vi "_Remote Connect.vi"(4 "error in (no error)":errorcluster, 7 "IP Address":string) -> (0 "error out":errorcluster, 3 "TCP":bool)   [LabVIEW 2015]
uses:
  Type/_RT Command.ctl
  Configuration/_Global Configuration.vi
  <vilib>/Utility/config.llb/Write Key (String).vi
  <vilib>/Utility/config.llb/NI_LVConfig.lvlib
panel:
  out "Info":string
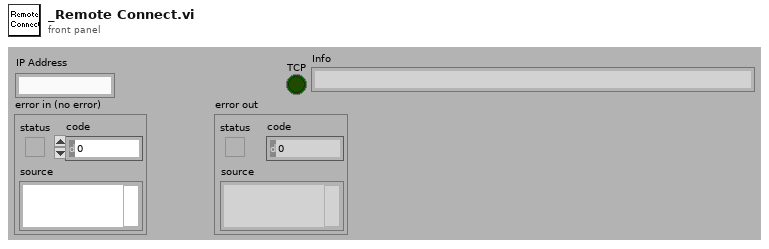
[diagram p1: front panel]
types:
  T1 = typedef "NI_LVConfig.lvlib/Config Data RefNum.ctl" = refnum<k1>
  T2 = typedef "_RT Command.ctl" = enum16{"xml Start Run", "xml Start Actual Run", "xml Stop Run", "xml Runtime Update", "xml Get Status", "xml Get Table", "xml Set Table", "xml Get Configuration", "xml System Status", "xml Set LC Input Logic", "xml Get Data", "xml Get Info", "Start", "StartActualRun", "Stop", "Runtime Update", "Get Data", "Get Info", "Get Status", "Get Param", "Get Config", "Get Table", "Read ADC", "Set Oscillator", "Update Config", "Update Table", "Set All Pol", "Set Pol and DC", "Set Max Mass", "Toggle RP", "Toggle EL", "Set PIC", "Initialize Turbo", "Send Turbo Comm", "Close Turbo", "P1", "P2", "P3", "Send Serial", "Set LC Out", "Get LC In", "Read VAC", "Test Table", "Toggle Power", "Get Startup", "Set Startup", "Get ADC Table", "Set ADC Table", "Get Brief Status", "Get Detail Status", "Auxiliary Update", "Set CC Logics", "Set CC Input Logics", "Ignore Error", "invalid"}
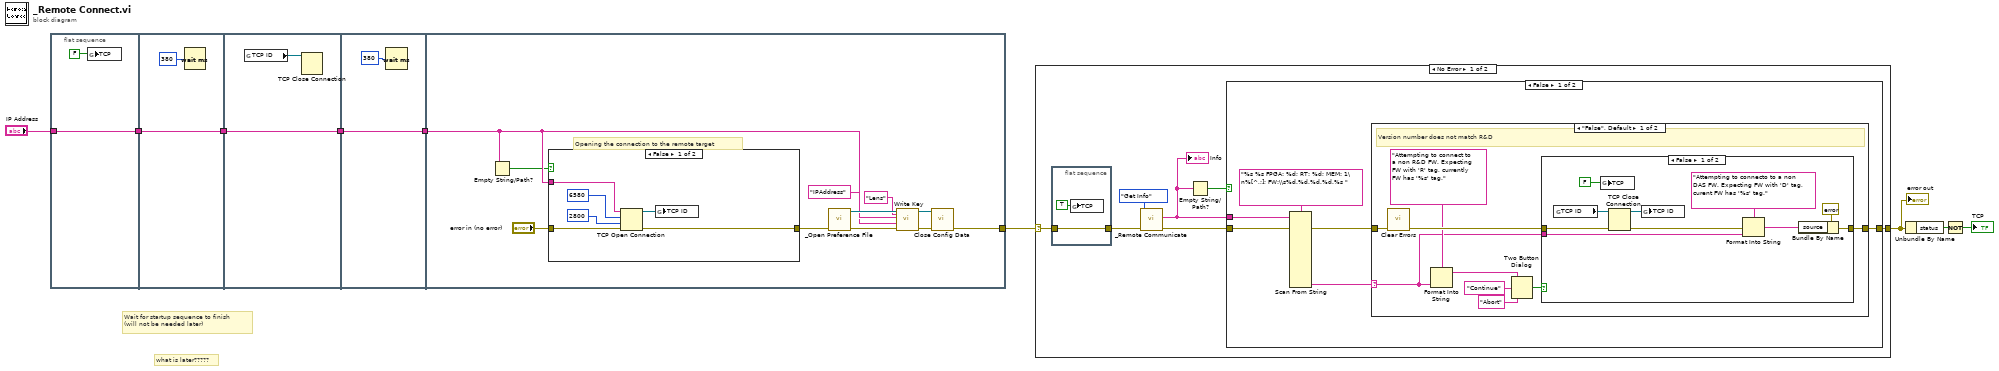
[diagram p0: block diagram]
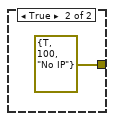
[diagram p2: hidden frame]
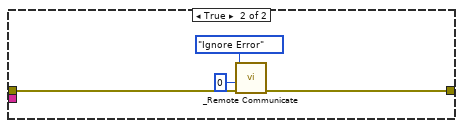
[diagram p3: hidden frame]
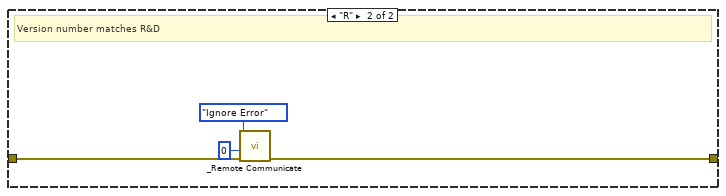
[diagram p4: hidden frame]
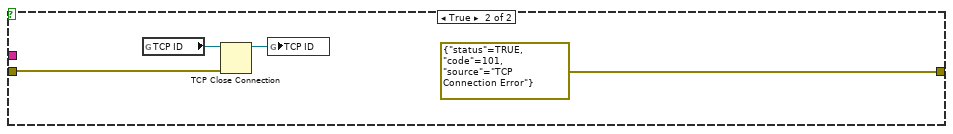
[diagram p5: hidden frame]
diagram:
  # "what is later?????"
  # "Wait for startup sequence to finish\n(will not be needed later)"
  n1 = flat-sequence {
    tunnel: "IP Address" -> [w10]
    tunnel: [w10] -> w4
    tunnel: w4 -> [w12]
    tunnel: [w12] -> w3
    tunnel: w3 -> [w14]
    tunnel: [w14] -> w2
    tunnel: w2 -> [w16]
    tunnel: [w16] -> w1
    tunnel: [w20] -> w9
    tunnel: w1 -> [w22]
    frame #0 {
      n2 = global write "_Global Configuration.vi" "TCP"(FALSE ("TCP")) -> ()
    }
    frame #1 {
      n3 = Wait (ms)(milliseconds to wait=u32 380) -> ()  [unwired: 1 out]
    }
    frame #2 {
      n4 = global read "_Global Configuration.vi" "TCP ID"() -> (w15:refnum<k5>)
      n5 = TCP Close Connection(connection ID=w15) -> ()  [unwired: 1 in, 3 out]
    }
    frame #3 {
      n6 = Wait (ms)(milliseconds to wait=u32 380) -> ()  [unwired: 1 out]
    }
    frame #4 {
      # "Opening the connection to the remote target"
      n7 = Empty String/Path?(string/path=w22) -> (empty?=w19:bool)
      n8 = case shown="False" w19 {
        tunnel: w22 -> [w33 _]
        tunnel: "error in (no error)" -> [w34 _]
        tunnel: [w30 errorcluster {"status"=TRUE, "code"=100, "source"="No IP"} ("error out")] -> w21
        frame False {
          n9 = TCP Open Connection(address=w33, remote port or service name=u16 6580 ("remote port"), timeout ms (60000)=2800, error in (no error)=w34) -> (connection ID=w31:refnum<k5>, error out=w30:errorcluster)  [unwired: 1 out]
          n10 = global write "_Global Configuration.vi" "TCP ID"(w31) -> ()
        }
        frame True {
        }
      }
      n11 = call "_Open Preference File.vi"("error In"=w21) -> ("error"=w26:errorcluster, "refnum"=w25:T1)  [unwired: 2 in, 3 out]
      n12 = call-poly <vilib>:"Write Key.vi"("section"="Lens", "error in (no error)"=w26, "value"=w22, "key"="IPAddress" ("section"), "refnum"=w25) -> ("error out"=w28:errorcluster, "refnum out"=w27:T1)  [unwired: 1 in, 4 out]
      n13 = call <vilib>:"Close Config Data.vi"("error in (no error)"=w28, "refnum"=w27) -> ("error out"=w20:errorcluster)  [unwired: 1 in, 8 out]
    }
  }
  n14 = case shown="No Error" w9 {
    selector: w9 -> [w41 w82]
    tunnel: [w38 w82] -> w7
    frame No Error {
      n15 = flat-sequence {
        tunnel: w41 -> [w80]
        tunnel: [w80] -> w40
        frame #0 {
          n16 = global write "_Global Configuration.vi" "TCP"(TRUE) -> ()
        }
      }
      n17 = call "_Remote Communicate.vi"("error in (no error)"=w40, "Command"=_RT_Command."Get Info") -> ("error out"=w39:errorcluster, "Info"=w36:string)  [unwired: 4 in, 2 out]
      "Info" <- w36
      n18 = Empty String/Path?(string/path=w36) -> (empty?=w37:bool)
      n19 = case shown="False" w37 {
        tunnel: w39 -> [w46 w78]
        tunnel: [w48 errorcluster {"status"=TRUE, "code"=101, "source"="TCP Connection Error"} ("error out")] -> w38
        tunnel: w36 -> [w43 _]
        frame False {
          n20 = Scan From String(format string="%s %s FPGA: %d; RT: %d; MEM: 1\n%[^,;]; FW:\\s%d.%d.%d.%d.%s ", input string=w43, error in=w46) -> (error out=w45:errorcluster, output 10=w44:string)  [unwired: 20 in, 2 out]
          n21 = case shown="\"False\", Default" w44 {
            selector: w44 -> [w49 _]
            tunnel: [w52 w73] -> w48
            tunnel: w45 -> [w57 w72]
            frame "False", Default {
              # "Version number does not match R&D"
              n22 = call <vilib>:"Clear Errors.vi"("error in (no error)"=w57) -> ("error out"=w53:errorcluster)  [unwired: 5 in, 1 out]
              n23 = Format Into String(format string="Attempting to connect to a non R&D FW. Expecting FW with 'R' tag, currently FW has '%s' tag." ("message"), w49) -> (resulting string=w50:string)  [unwired: 2 in, 1 out]
              n24 = Two Button Dialog(message=w50, 1:"Abort" ("F button name (\"Cancel\")"), 2:"Continue" ("T button name (\"OK\")")) -> (T button?=w54:bool)
              n25 = case shown="False" w54 {
                tunnel: w53 -> [w65 w68]
                tunnel: [w59 w69] -> w52
                tunnel: w49 -> [w61 _]
                frame False {
                  n26 = global read "_Global Configuration.vi" "TCP ID"() -> (w67:refnum<k5>)
                  n27 = global write "_Global Configuration.vi" "TCP"(FALSE) -> ()
                  n28 = TCP Close Connection(connection ID=w67, error in (no error)=w65) -> (connection ID out=w66:refnum<k5>, error out=w60:errorcluster)  [unwired: 1 in]
                  n29 = global write "_Global Configuration.vi" "TCP ID"(w66) -> ()
                  n30 = Format Into String(format string="Attempting to connecto to a non DAS FW. Expecting FW with 'D' tag, curent FW has '%s' tag." ("source"), error in=w60, w61) -> (resulting string=w62:string)  [unwired: 1 in, 1 out]
                  n31 = Bundle By Name(cluster=errorcluster {"status"=TRUE, "code"=110, "source"="Attempting to connecto to a non MD FW"} ("error out"), "source"=w62) -> (w59:errorcluster)
                }
                frame True {
                  n32 = call "_Remote Communicate.vi"("error in (no error)"=w68, "DC Param"=u16 0, "Command"=_RT_Command."Ignore Error") -> ("error out"=w69:errorcluster)  [unwired: 3 in, 3 out]
                }
              }
            }
            frame "R" {
              # "Version number matches R&D"
              n33 = call "_Remote Communicate.vi"("error in (no error)"=w72, "DC Param"=u16 0, "Command"=_RT_Command."Ignore Error") -> ("error out"=w73:errorcluster)  [unwired: 3 in, 3 out]
            }
          }
        }
        frame True {
          n34 = global read "_Global Configuration.vi" "TCP ID"() -> (w77:refnum<k5>)
          n35 = TCP Close Connection(connection ID=w77, error in (no error)=w78) -> (connection ID out=w76:refnum<k5>)  [unwired: 1 in, 1 out]
          n36 = global write "_Global Configuration.vi" "TCP ID"(w76) -> ()
        }
      }
    }
    frame Error {
    }
  }
  "error out" <- w7
  n37 = Unbundle By Name(w7) -> ("status"=w8:bool)
  n38 = Not(x=w8) -> (.not. x?=→"TCP":bool)
